vi "Test FGen API.vi"() -> ()   [LabVIEW 2020]
doc: "FGen API Tester."
uses:
  FGen.lvlib
panel:
  in  "Set Generator Type":bool
  in  "Funciones":string(combo)
  out "Signal":waveform(dbl)(graph)
  in  "Generate Signal":bool
  in  "Set to Default":bool
  in  "signal type":T1(ring)
  in  "Set Signal Type":bool
  in  "Run as Singleton?":bool
  in  "Show Block Diagram":bool
  in  "Refresh Modules":bool
  out "Active Modules":string[](array[string])
  in  "Stop Module":bool
  in  "Select Module":i32(ring)=-1 caption="Select Module\nTo send Request to" items=["All"=-1]
  in  "Run New Module":bool
  in  "Hide Module Panel":bool
  in  "Show Module Panel":bool
  out "Status":string
  # "This VI tests the API for the Module."
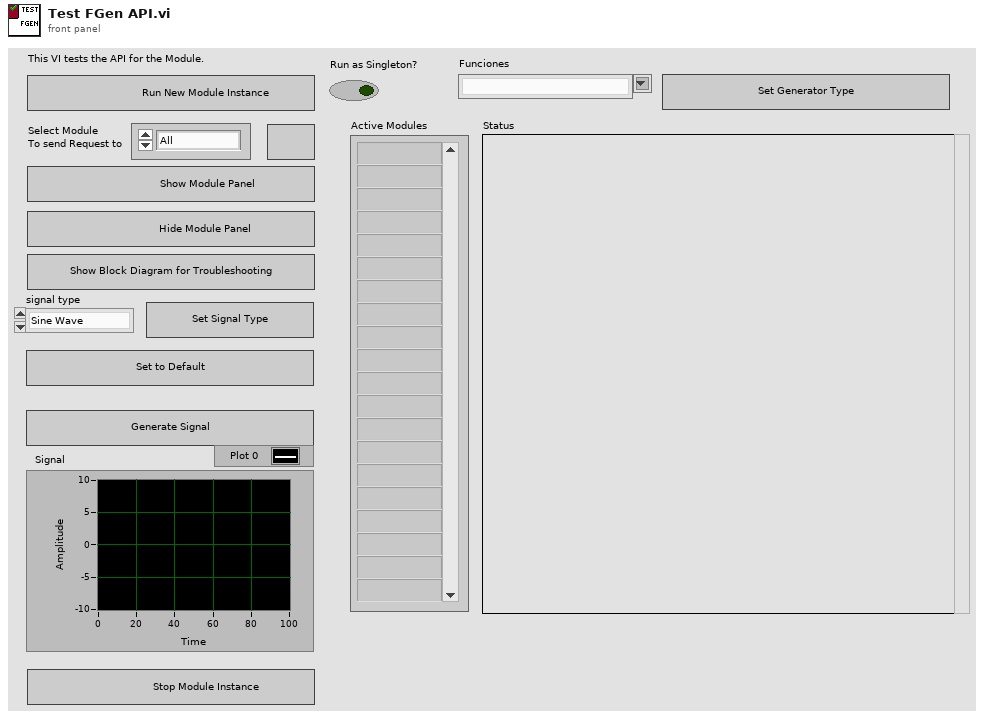
[diagram p1: front panel]
types:
  T1 = enum16{"Sine Wave", "Triangle Wave", "Square Wave", "Sawtooth Wave"}
  T2 = typedef "FGen.lvlib/Broadcast Events--cluster.ctl" = cluster{"Module Did Init":refnum<user-event>, "Status Updated":refnum<user-event>, "Error Reported":refnum<user-event>, "Module Did Stop":refnum<user-event>, "Update Module Execution Status":refnum<user-event>, "Type_Function":refnum<user-event>}
  T3 = typedef "FGen.lvlib/Generate Signal (Reply Payload)--cluster.ctl" = cluster{"signal out":waveform(dbl), "Generate Signal_error":errorcluster}
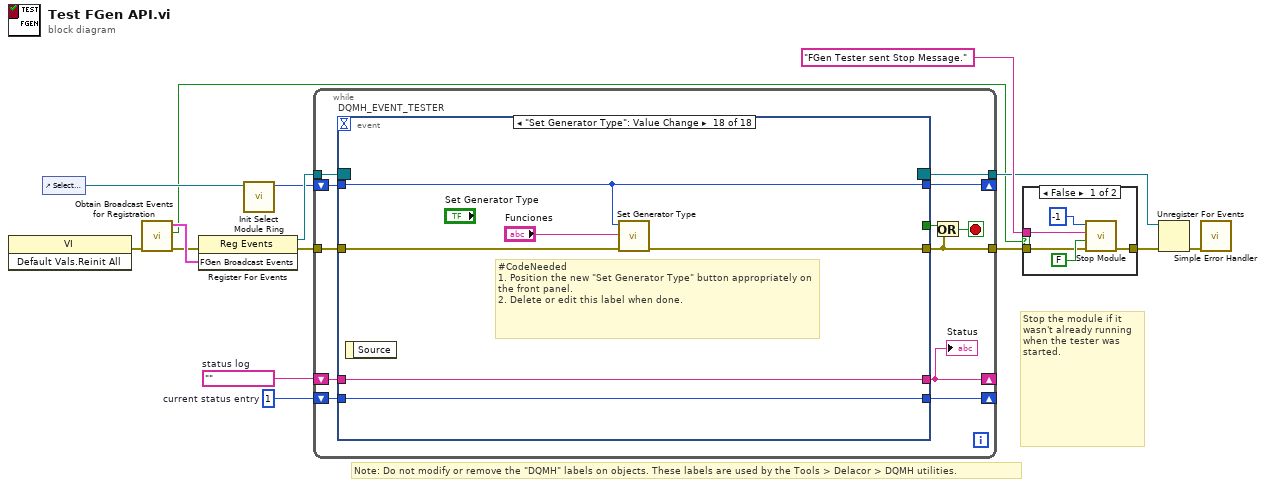
[diagram p0: block diagram]
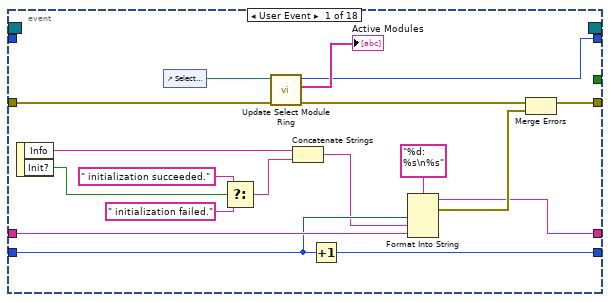
[diagram p3: hidden frame]
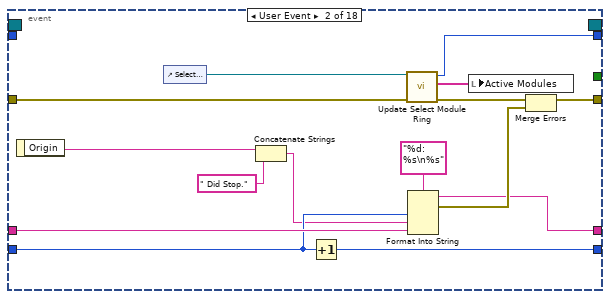
[diagram p4: hidden frame]
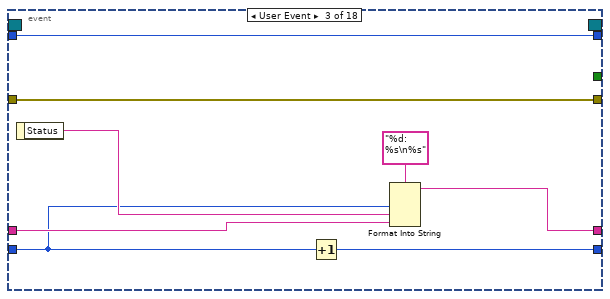
[diagram p5: hidden frame]
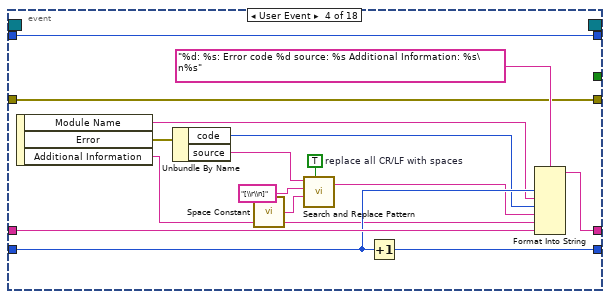
[diagram p6: hidden frame]
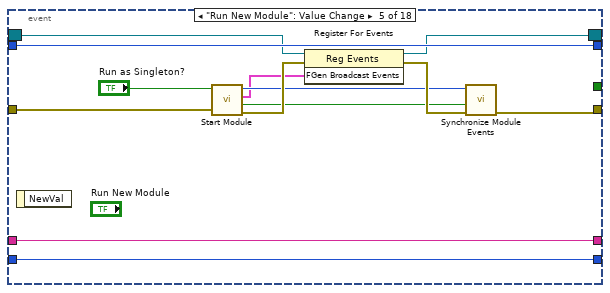
[diagram p7: hidden frame]
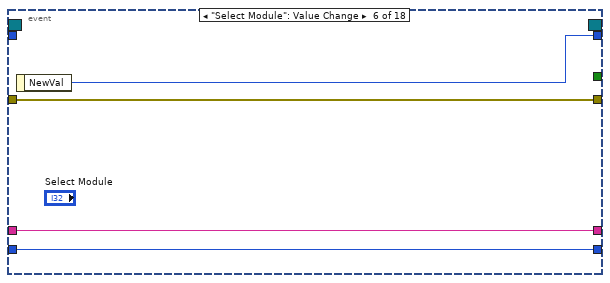
[diagram p8: hidden frame]
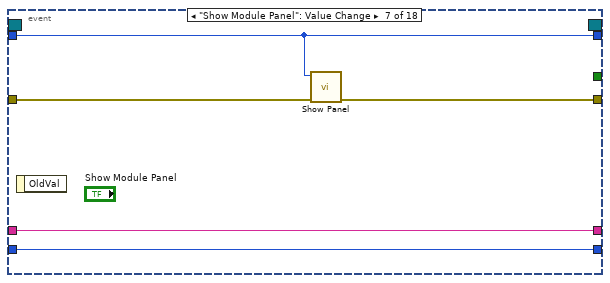
[diagram p9: hidden frame]
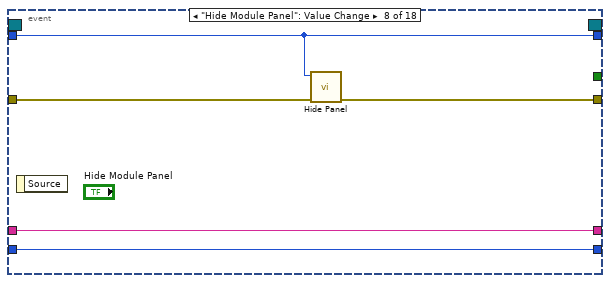
[diagram p10: hidden frame]
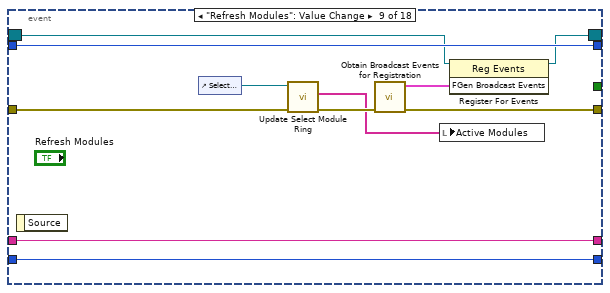
[diagram p11: hidden frame]
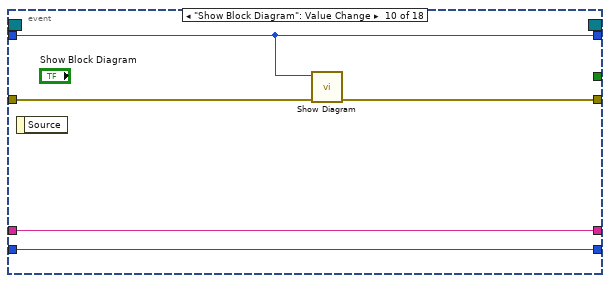
[diagram p12: hidden frame]
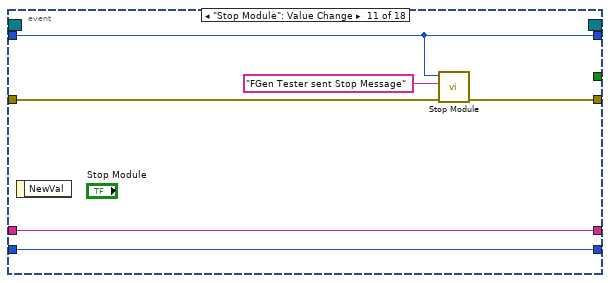
[diagram p13: hidden frame]
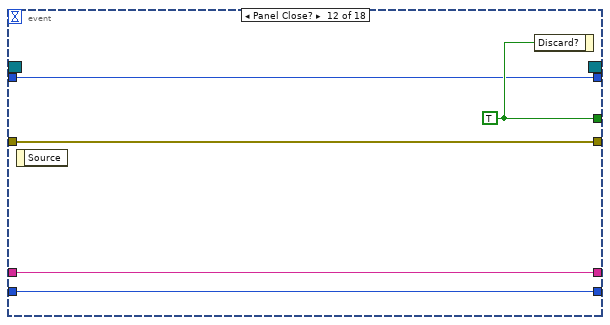
[diagram p14: hidden frame]
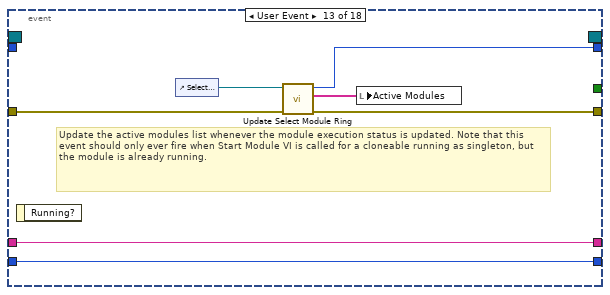
[diagram p15: hidden frame]
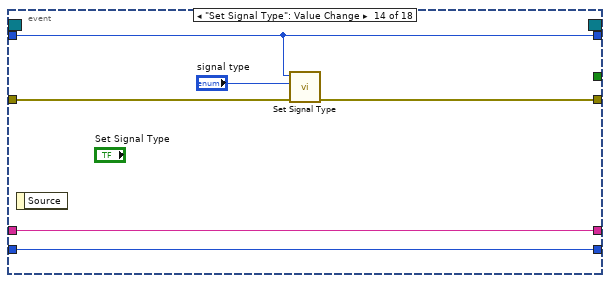
[diagram p16: hidden frame]
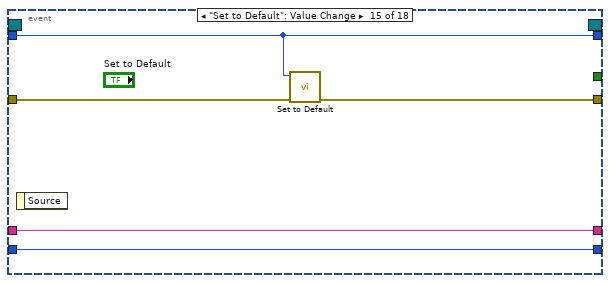
[diagram p17: hidden frame]
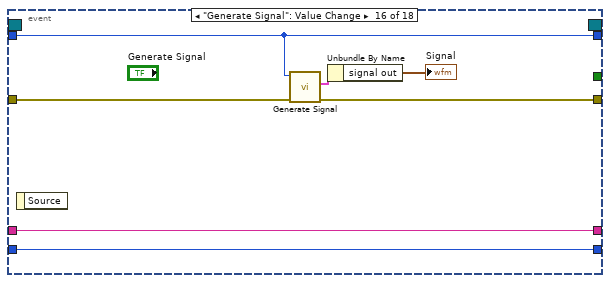
[diagram p18: hidden frame]
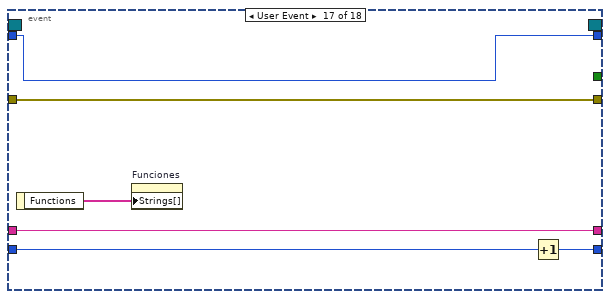
[diagram p19: hidden frame]
diagram:
  w12 = 1  # current status entry
  w13 = ""  # status log
  # "Stop the module if it wasn't already running when the tester was started."
  # "Note: Do not modify or remove the \"DQMH\" labels on objects. These labels are used by the Tools > Delacor > DQMH utilities."
  n1 = invoke class="VI" method="Default Vals.Reinit All"() -> (error out=w5:errorcluster)  [unwired: 3 in, 2 out]
  n2 = control-ref of="Select Module"() -> (w10:refnum<vi>)
  n3 = call "Obtain Broadcast Events for Registration.vi"("error in (no error)"=w5) -> ("error out"=w4:errorcluster, "Already running?"=w3:bool, "FGen Broadcast Events"=w9:T2)  [unwired: 8 in]
  n4 = register-events(error in=w4, w9) -> (reference out=w15:refnum<event-registration>, error out=w8:errorcluster)  [unwired: 1 in]
  n5 = call "Init Select Module Ring.vi"("Select Module Ring Ref"=w10) -> ("Value for All Modules"=w11:i32)  [unwired: 8 in, 2 out]
  n6 = while {
    tunnel: w15 -> [w27]
    tunnel: [w16] -> w2
    tunnel: w8 -> [w25]
    shift-right: [w21] -> _
    shift-left: w13 -> [w23]
    shift-right: [w22] -> _
    shift-left: w12 -> [w24]
    shift-right: [w18] -> _
    shift-left: w11 -> [w19]
    tunnel: [w17] -> w6
    stop <- w20 stop-if-true
    n7 = event "DQMH_EVENT_TESTER" shown="[17] \"Set Generator Type\": Value Change" {
      selector: w27 -> [_ _ _ _ w91 _ _ _ w117 _ _ _ _ _ _ _ _ _]
      dyn-events: [_ _ _ _ w90 _ _ _ w116 _ _ _ _ _ _ _ _ _] -> w17
      timeout: _ -> [_ _ _ _ _ _ _ _ _ _ _ _ _ _ _ _ _ _]
      tunnel: [_ _ _ _ _ _ _ _ _ _ _ w138 _ _ _ _ _ _] -> w26
      tunnel: [w35 w52 w68 w74 w89 w101 w105 w110 w113 w124 w129 w137 w141 w148 w153 w160 w169 w172] -> w16
      tunnel: w25 -> [w37 w54 w68 w74 w92 w101 w106 w111 w118 w127 w130 w137 w142 w151 w156 w163 w169 w175]
      tunnel: w24 -> [w42 w57 w61 w80 w94 w99 w103 w108 w121 w125 w132 w135 w144 w149 w154 w161 w167 w173]
      tunnel: w23 -> [w43 w58 w64 w82 w95 w100 w104 w109 w122 w126 w133 w136 w145 w150 w155 w162 w165 w174]
      tunnel: [w40 w55 w65 w77 w95 w100 w104 w109 w122 w126 w133 w136 w145 w150 w155 w162 w165 w174] -> w21
      tunnel: [w41 w56 w67 w83 w94 w99 w103 w108 w121 w125 w132 w135 w144 w149 w154 w161 w166 w173] -> w22
      tunnel: w19 -> [_ _ w62 w84 w93 _ w102 w107 w120 w123 w131 w134 _ w147 w152 w159 w168 w170]
      tunnel: [w32 w49 w62 w84 w93 w98 w102 w107 w120 w123 w131 w134 w140 w147 w152 w159 w168 w170] -> w18
      event User Event {
        n8 = event-data() -> ("Info"=w39:string, "Init?"=w29:bool)  [unwired: 1 in]
        n9 = control-ref of="Select Module"() -> (w34:refnum<vi>)
        n10 = Select(t=" initialization succeeded.", s=w29, f=" initialization failed.") -> (s? t:f=w28:string)
        n11 = call "Update Select Module Ring.vi"("error in (no error)"=w37, "Select Module Ring Ref"=w34) -> ("error out"=w36:errorcluster, "Active Modules (Array)"=→"Active Modules":string[], "New Module Ring Value"=w32:i32)  [unwired: 7 in]
        n12 = Concatenate Strings(w39, w28) -> (w38:string)
        n13 = Increment(x=w42) -> (x+1=w41:i32)
        n14 = Format Into String(format string="%d: %s\n%s", w42, w38, w43) -> (resulting string=w40:string, error out=w45:errorcluster)  [unwired: 2 in]
        n15 = Merge Errors(w36, w45) -> (w35:errorcluster)
      }
      event User Event {
        n16 = event-data() -> ("Origin"=w47:string)  [unwired: 1 in]
        n17 = control-ref of="Select Module"() -> (w51:refnum<vi>)
        n18 = Concatenate Strings(w47, " Did Stop.") -> (w46:string)
        n19 = Increment(x=w57) -> (x+1=w56:i32)
        n20 = call "Update Select Module Ring.vi"("error in (no error)"=w54, "Select Module Ring Ref"=w51) -> ("error out"=w53:errorcluster, "Active Modules (Array)"=w50:string[], "New Module Ring Value"=w49:i32)  [unwired: 7 in]
        n21 = Format Into String(format string="%d: %s\n%s", w57, w46, w58) -> (resulting string=w55:string, error out=w60:errorcluster)  [unwired: 2 in]
        n22 = local write "Active Modules"(w50) -> ()
        n23 = Merge Errors(w53, w60) -> (w52:errorcluster)
      }
      event User Event {
        n24 = event-data() -> ("Status"=w63:string)  [unwired: 1 in]
        n25 = Increment(x=w61) -> (x+1=w67:i32)
        n26 = Format Into String(format string="%d: %s\n%s", w61, w63, w64) -> (resulting string=w65:string)  [unwired: 2 in, 1 out]
      }
      event User Event {
        w78 = TRUE  # replace all CR/LF with spaces
        n27 = event-data() -> ("Module Name"=w72:string, "Error"=w71:errorcluster, "Additional Information"=w69:string)  [unwired: 1 in]
        n28 = Unbundle By Name(w71) -> ("code"=w73:i32, "source"=w75:string)
        n29 = call <vilib>:"Space Constant.vi"() -> ("String"=w79:string)
        n30 = call <vilib>:"Search and Replace Pattern.vi"("string"=w75, "regular expression (\"\")"="[\\r\\n]" ("regular expression (\"\")"), "replace string (\"\")"=w79, "replace all? (F)"=w78) -> ("result string"=w76:string)  [unwired: 1 in, 1 out]
        n31 = Increment(x=w80) -> (x+1=w83:i32)
        n32 = Format Into String(format string="%d: %s: Error code %d source: %s Additional Information: %s\n%s", w80, w72, w73, w76, w69, w82) -> (resulting string=w77:string)  [unwired: 2 in, 1 out]
      }
      event "Run New Module": Value Change {
        n33 = event-data() -> ()  [unwired: 1 in, 1 out]
        n34 = call "Start Module.vi"("error in"=w92, "Run as Singleton? (F)"="Run as Singleton?") -> ("error out"=w96:errorcluster, "Wait for Event Sync?"=w87:bool, "FGen Broadcast Events"=w86:T2, "Module ID"=w88:i32)  [unwired: 6 in]
        n35 = register-events(reference=w91, error in=w96, w86) -> (reference out=w90:refnum<event-registration>, error out=w97:errorcluster)
        n36 = call "Synchronize Module Events.vi"("error in"=w97, "Wait for Event Sync?"=w87, "Module ID in"=w88) -> ("error out"=w89:errorcluster)  [unwired: 7 in, 1 out]
      }
      event "Select Module": Value Change {
        n37 = event-data() -> ("NewVal"=w98:i32)  [unwired: 1 in]
      }
      event "Show Module Panel": Value Change {
        n38 = event-data() -> ()  [unwired: 1 in, 1 out]
        n39 = call "Show Panel.vi"("error in (no error)"=w106, "Module ID"=w102) -> ("error out"=w105:errorcluster)  [unwired: 9 in]
      }
      event "Hide Module Panel": Value Change {
        n40 = event-data() -> ()  [unwired: 1 in, 1 out]
        n41 = call "Hide Panel.vi"("error in (no error)"=w111, "Module ID"=w107) -> ("error out"=w110:errorcluster)  [unwired: 9 in]
      }
      event "Refresh Modules": Value Change {
        n42 = event-data() -> ()  [unwired: 1 in, 1 out]
        n43 = control-ref of="Select Module"() -> (w119:refnum<vi>)
        n44 = call "Update Select Module Ring.vi"("error in (no error)"=w118, "Select Module Ring Ref"=w119) -> ("error out"=w114:errorcluster, "Active Modules (Array)"=w112:string[])  [unwired: 7 in, 1 out]
        n45 = call "Obtain Broadcast Events for Registration.vi"("error in (no error)"=w114) -> ("error out"=w113:errorcluster, "FGen Broadcast Events"=w115:T2)  [unwired: 8 in, 1 out]
        n46 = local write "Active Modules"(w112) -> ()
        n47 = register-events(reference=w117, w115) -> (reference out=w116:refnum<event-registration>)  [unwired: 1 in, 1 out]
      }
      event "Show Block Diagram": Value Change {
        n48 = event-data() -> ()  [unwired: 1 in, 1 out]
        n49 = call "Show Diagram.vi"("error in (no error)"=w127, "Module ID"=w123) -> ("error out"=w124:errorcluster)  [unwired: 9 in]
      }
      event "Stop Module": Value Change {
        n50 = event-data() -> ()  [unwired: 1 in, 1 out]
        n51 = call "Stop Module.vi"("error in (no error)"=w130, "Origin"="FGen Tester sent Stop Message", "Module ID"=w131) -> ("error out"=w129:errorcluster)  [unwired: 8 in]
      }
      event Panel Close? {
        w138 = TRUE ("Discard?")
        n52 = event-data() -> ()  [unwired: 1 in, 1 out]
        n53 = event-data("Discard?"=w138) -> ()  [unwired: 1 in, 1 out]
      }
      event User Event {
        # "Update the active modules list whenever the module execution status is updated. Note that this event should only ever fire when Start Module VI is called for a cloneable running as singleton, but the module is already running."
        n54 = event-data() -> ()  [unwired: 1 in, 1 out]
        n55 = control-ref of="Select Module"() -> (w143:refnum<vi>)
        n56 = call "Update Select Module Ring.vi"("error in (no error)"=w142, "Select Module Ring Ref"=w143) -> ("error out"=w141:errorcluster, "Active Modules (Array)"=w139:string[], "New Module Ring Value"=w140:i32)  [unwired: 7 in]
        n57 = local write "Active Modules"(w139) -> ()
      }
      event "Set Signal Type": Value Change {
        n58 = event-data() -> ()  [unwired: 1 in, 1 out]
        n59 = call "Set Signal Type.vi"("error in"=w151, "signal type"="signal type", "Module ID"=w147) -> ("error out"=w148:errorcluster)  [unwired: 8 in]
      }
      event "Set to Default": Value Change {
        n60 = event-data() -> ()  [unwired: 1 in, 1 out]
        n61 = call "Set to Default.vi"("error in"=w156, "Module ID"=w152) -> ("error out"=w153:errorcluster)  [unwired: 9 in]
      }
      event "Generate Signal": Value Change {
        n62 = event-data() -> ()  [unwired: 1 in, 1 out]
        n63 = call "Generate Signal.vi"("error in"=w163, "Module ID"=w159) -> ("error out"=w160:errorcluster, "Reply Payload"=w158:T3)  [unwired: 7 in, 1 out]
        n64 = Unbundle By Name(w158) -> ("signal out"=→"Signal":waveform(dbl))
      }
      event User Event {
        n65 = event-data() -> ("Functions"=w164:string[])  [unwired: 1 in]
        n66 = property on="Funciones" class="CmbBox"("Strings[]"=w164) -> ()  [unwired: 2 in, 2 out]
        n67 = Increment(x=w167) -> (x+1=w166:i32)
      }
      event "Set Generator Type": Value Change {
        # "#CodeNeeded\n1. Position the new \"Set Generator Type\" button appropriately on the front panel.\n2. Delete or edit this label when done."
        n68 = event-data() -> ()  [unwired: 1 in, 1 out]
        n69 = call "Set Generator Type.vi"("error in"=w175, "Funcion"="Funciones", "Module ID"=w170) -> ("error out"=w172:errorcluster)  [unwired: 8 in]
      }
    }
    "Status" <- w21
    n70 = Or(x=w26, y=w16) -> (x .or. y?=w20:bool)
  }
  n71 = case shown="False" w3 {
    tunnel: [w180 w181] -> w14
    tunnel: "FGen Tester sent Stop Message." ("Origin") -> [w179 _]
    tunnel: w2 -> [w176 w181]
    frame False {
      n72 = call "Stop Module.vi"("error in (no error)"=w176, "Wait for Module to stop? (F)"=FALSE ("Wait for Module to stop?"), "Origin"=w179, "Module ID"=-1 ("Stop all")) -> ("error out"=w180:errorcluster)  [unwired: 7 in]
    }
    frame True {
    }
  }
  n73 = Unregister For Events(event registration refnum=w6, error in=w14) -> (error out=w1:errorcluster)
  n74 = call <vilib>:"Simple Error Handler.vi"("error in (no error)"=w1) -> ()  [unwired: 4 in, 5 out]
